vi "Object Layout Classes.vi"(7 "application reference":refnum<vi>, 8 "error in":errorcluster, 10 "rescan (F)":bool) -> (0 "error out":errorcluster, 3 "object layout classes":refnum<class "Object Layout.lvclass">[](array[class]))   [LabVIEW 2010, in "NI_SE_Front Panel Layout.lvlib"]
uses:
  NI_SE_Front Panel Layout.lvlib
  Object Layout Classes/Object Layout/Object Layout.lvclass
  Object Layout Classes/Ring Layout/Ring Layout.lvclass
  Object Layout Classes/Decoration Layout/Decoration Layout.lvclass
  Object Layout Classes/Slide Control Layout/Slide Control Layout.lvclass
  Object Layout Classes/Knob Control Layout/Knob Control Layout.lvclass
  Object Layout Classes/NumericWithScale Control Layout/NumericWithScale Control Layout.lvclass
  Object Layout Classes/XControl Layout/XControl Layout.lvclass
  Object Layout Classes/Subpanel Control Layout/Subpanel Control Layout.lvclass
  Object Layout Classes/Tree Control Layout/Tree Control Layout.lvclass
  Object Layout Classes/String Control Layout/String Control Layout.lvclass
  Object Layout Classes/Tab Control Layout/Tab Control Layout.lvclass
  Object Layout Classes/GraphChart Control Layout/GraphChart Control Layout.lvclass
  Object Layout Classes/Listbox Control Layout/Listbox Control Layout.lvclass
  Object Layout Classes/NamedNumeric Control Layout/NamedNumeric Control Layout.lvclass
  Object Layout Classes/Digital Control Layout/Digital Control Layout.lvclass
  Object Layout Classes/Boolean Control Layout/Boolean Control Layout.lvclass
  Object Layout Classes/Splitter Layout/Splitter Layout.lvclass
  Object Layout Classes/Pane Layout/Pane Layout.lvclass
  Object Layout Classes/Cluster Control Layout/Cluster Control Layout.lvclass
  Object Layout Classes/Array Control Layout/Array Control Layout.lvclass
  Object Layout Classes/Text Decoration Layout/Text Decoration Layout.lvclass
  Object Layout Classes/Control Layout/Control Layout.lvclass
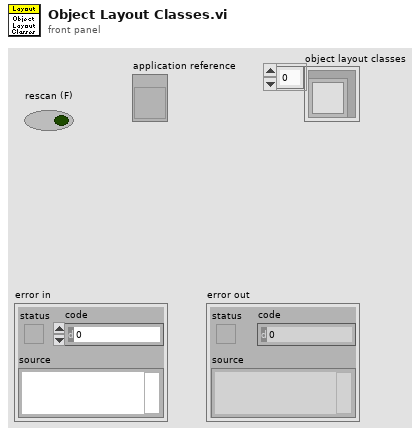
[diagram p1: front panel]
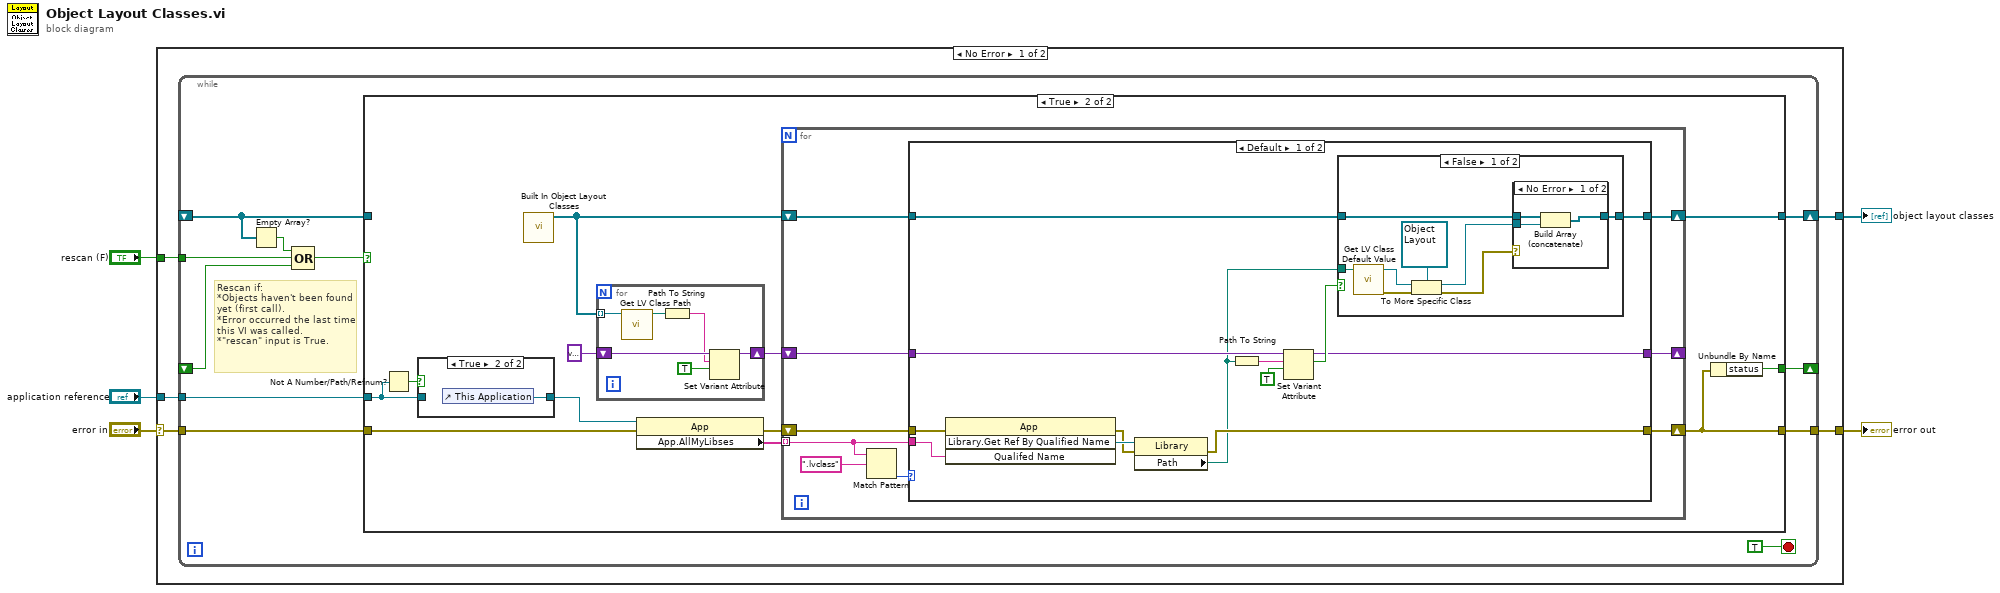
[diagram p0: block diagram]
diagram:
  n1 = case shown="No Error" "error in" {
    selector: "error in" -> [w10 w82]
    tunnel: "rescan (F)" -> [w9 _]
    tunnel: [w8 w82] -> w3
    tunnel: [w7 _] -> w2
    tunnel: "application reference" -> [w6 _]
    frame No Error {
      n2 = while {
        tunnel: w10 -> [w21]
        tunnel: [w20] -> w8
        tunnel: w9 -> [w18]
        shift-right: [w19] -> w7
        shift-left: _ -> [w15]
        shift-right: [w13] -> _
        shift-left: _ -> [w12]
        tunnel: w6 -> [w11]
        stop <- TRUE stop-if-true
        # "Rescan if:\n*Objects haven't been found yet (first call).\n*Error occurred the last time this VI was called.\n*\"rescan\" input is True."
        n3 = Empty Array?(array=w15) -> (empty?=w14:bool)
        n4 = Compound Arithmetic op=OR(w14, w18, w12) -> (w17:bool)
        n5 = case shown="True" w17 {
          tunnel: w21 -> [w23 w35]
          tunnel: [w23 w29] -> w20
          tunnel: [w22 w30] -> w19
          tunnel: w15 -> [w22 _]
          tunnel: [_ w28] -> w13
          tunnel: w11 -> [_ w25]
          frame False {
            # "Classes have already been scanned."
          }
          frame True {
            n6 = Not A Number/Path/Refnum?(number/path/refnum=w25) -> (NaN/Path/Refnum?=w26:bool)
            n7 = case shown="True" w26 {
              tunnel: [w36 w37] -> w24
              tunnel: w25 -> [w36 _]
              frame False {
              }
              frame True {
                n8 = control-ref of="This Application"() -> (w37:refnum<vi>)
              }
            }
            n9 = call "Built In Object Layout Classes.vi"() -> ("built in object layout classes"=w27:refnum<class "Object Layout.lvclass">[])  [unwired: 10 in, 1 out]
            n10 = for {
              tunnel: w27 -> [w43] mode=indexing
              shift-right: [w42] -> w31
              shift-left: variant -> [w40]
              n11 = call <vilib>:"Get LV Class Path.vi"("object"=w43) -> ("class path"=w39:path)  [unwired: 9 in, 1 out]
              n12 = Path To String(path=w39) -> (string=w38:string)
              n13 = Set Variant Attribute(Variant=w40, name=w38, value=TRUE) -> (Variant out=w42:variant)  [unwired: 1 in, 2 out]
            }
            n14 = property class="App"(reference=w24, error in=w35) -> (error out=w34:errorcluster, "App.AllMyLibses"=w33:string[])  [unwired: 1 out]
            n15 = for {
              shift-right: [w51] -> w30
              shift-left: w27 -> [w52]
              shift-right: [w47] -> w29
              shift-left: w34 -> [w48]
              tunnel: w33 -> [w46] mode=indexing
              shift-right: [w44] -> _
              shift-left: w31 -> [w45]
              n16 = Match Pattern(string=w46, regular expression=".lvclass") -> (offset past match=w49:i32)  [unwired: 1 in, 3 out]
              n17 = case shown="Default" w49 {
                tunnel: w52 -> [w65 w81]
                tunnel: [w64 w81] -> w51
                tunnel: w48 -> [w63 w80]
                tunnel: [w59 w80] -> w47
                tunnel: w46 -> [w62 _]
                tunnel: w45 -> [w58 w79]
                tunnel: [w55 w79] -> w44
                frame Default {
                  n18 = invoke class="App" method="Library.Get Ref By Qualified Name"(error in=w63, "Qualifed Name"=w62) -> (error out=w60:errorcluster, "Library.Get Ref By Qualified Name"=w61:refnum<vi>)  [unwired: 2 in, 2 out]
                  n19 = property class="Library"(reference=w61, error in=w60) -> (error out=w59:errorcluster, "Path"=w54:path)  [unwired: 1 out]
                  n20 = Path To String(path=w54) -> (string=w53:string)
                  n21 = Set Variant Attribute(Variant=w58, name=w53, value=TRUE) -> (Variant out=w55:variant, replaced=w56:bool)  [unwired: 1 in, 1 out]
                  n22 = case shown="False" w56 {
                    tunnel: w65 -> [w69 w78]
                    tunnel: [w68 w78] -> w64
                    tunnel: w54 -> [w67 _]
                    frame False {
                      n23 = call <vilib>:"Get LV Class Default Value.vi"("class path"=w67) -> ("error out"=w73:errorcluster, "object"=w72:refnum<class>)  [unwired: 9 in]
                      n24 = To More Specific Class(target class=refnum<class "Object Layout.lvclass"> refnum ("NI_SE_Front Panel Layout.lvlib:Object Layout.lvclass"), reference=w72, error in=w73) -> (specific class reference=w70:refnum<class "Object Layout.lvclass">, error out=w66:errorcluster)
                      n25 = case shown="No Error" w66 {
                        tunnel: w69 -> [w76 w77]
                        tunnel: w70 -> [w75 _]
                        tunnel: [w74 w77] -> w68
                        frame No Error {
                          n26 = Build Array (concatenate)(w76, w75) -> (w74:refnum<class "Object Layout.lvclass">[])
                        }
                        frame Error {
                        }
                      }
                    }
                    frame True {
                      # "Class is already in the array."
                    }
                  }
                }
                frame -1 {
                  # "Library is not a class."
                }
              }
            }
            n27 = Unbundle By Name(w29) -> ("status"=w28:bool)
          }
        }
      }
    }
    frame Error {
    }
  }
  "object layout classes" <- w2
  "error out" <- w3
